vi "Day 16-Unpack Operator.vi"(11 "String in":string) -> (1 "Results Array":u64[](array[numeric]), 2 "Sum of Versions":u64, 3 "String out":string)   [LabVIEW 2021]
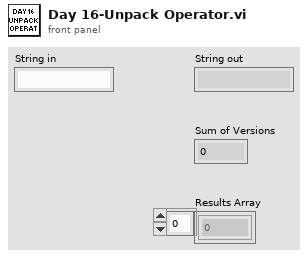
[diagram p1: front panel]
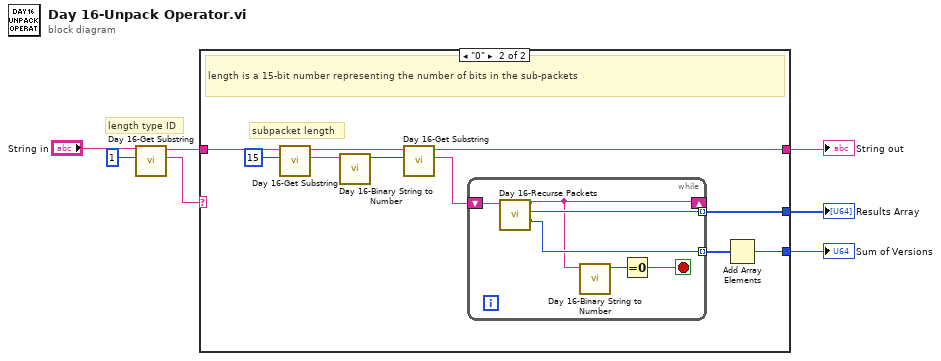
[diagram p0: block diagram]
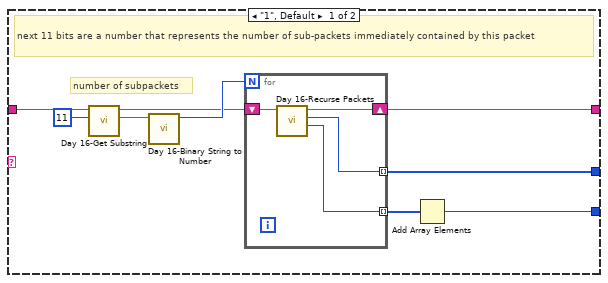
[diagram p2: hidden frame]
diagram:
  # "length type ID"
  n1 = call "Day 16-Get Substring.vi"("length"=1, "String in"="String in") -> ("Substring"=w4:string, "String out"=w3:string)  [unwired: 8 in]
  n2 = case shown="\"0\"" w4 {
    tunnel: w3 -> [w15 w29]
    tunnel: [w12 w27] -> w5
    tunnel: [w10 w24] -> w6
    tunnel: [w8 w23] -> w7
    frame "1", Default {
      # "number of subpackets"
      # "next 11 bits are a number that represents the number of sub-packets immediately contained by this packet"
      n3 = call "Day 16-Get Substring.vi"("length"=11, "String in"=w15) -> ("Substring"=w11:string, "String out"=w13:string)  [unwired: 8 in]
      n4 = call "Day 16-Binary String to Number.vi"("Substring"=w11) -> ("Numeric"=w14:u64)  [unwired: 10 in]
      n5 = for {
        N: w14 -> [_]
        shift-right: [w19] -> w12
        shift-left: w13 -> [w20]
        tunnel: [w18] -> w9 mode=indexing
        tunnel: [w17] -> w8 mode=indexing
        n6 = call "Day 16-Recurse Packets.vi"("String"=w20) -> ("Sum of Versions"=w18:u64, "Return Value"=w17:u64, "Left over bits"=w19:string)  [unwired: 8 in]
      }
      n7 = Add Array Elements(numeric array=w9) -> (sum=w10:u64)
    }
    frame "0" {
      # "subpacket length"
      # "length is a 15-bit number representing the number of bits in the sub-packets"
      n8 = call "Day 16-Get Substring.vi"("length"=15, "String in"=w29) -> ("Substring"=w22:string, "String out"=w28:string)  [unwired: 8 in]
      n9 = call "Day 16-Binary String to Number.vi"("Substring"=w22) -> ("Numeric"=w21:u64)  [unwired: 10 in]
      n10 = call "Day 16-Get Substring.vi"("length"=w21, "String in"=w28) -> ("Substring"=w26:string, "String out"=w27:string)  [unwired: 8 in]
      n11 = while {
        tunnel: [w34] -> w25 mode=indexing
        shift-right: [w32] -> _
        shift-left: w26 -> [w36]
        tunnel: [w33] -> w23 mode=indexing
        stop <- w35 stop-if-true
        n12 = call "Day 16-Recurse Packets.vi"("String"=w36) -> ("Sum of Versions"=w34:u64, "Return Value"=w33:u64, "Left over bits"=w32:string)  [unwired: 8 in]
        n13 = call "Day 16-Binary String to Number.vi"("Substring"=w32) -> ("Numeric"=w31:u64)  [unwired: 10 in]
        n14 = Equal To 0?(x=w31) -> (x = 0?=w35:bool)
      }
      n15 = Add Array Elements(numeric array=w25) -> (sum=w24:u64)
    }
  }
  "Results Array" <- w7
  "Sum of Versions" <- w6
  "String out" <- w5
